vi "Add State (to Connections).vi"(8 "error in (no error)":errorcluster, 10 "State":string, 11 "Channel Ref in":T1 format="%.0x") -> (0 "error out":errorcluster, 3 "Channel Ref out":T1=18446744073709551615 format="%.0x")   [LabVIEW 2017, in "Switch Scripting.lvlib"]
uses:
  Switch Scripting.lvlib
  <vilib>/NI Veristand/Custom Device API/Custom Device Item Ref.ctl
  NationalInstruments.VeriStand.SystemDefinitionAPI
  Shared/Constants.vi
  Shared/Switch Shared.lvlib
  <vilib>/NI VeriStand/Custom Device API/Custom Device API.lvlib
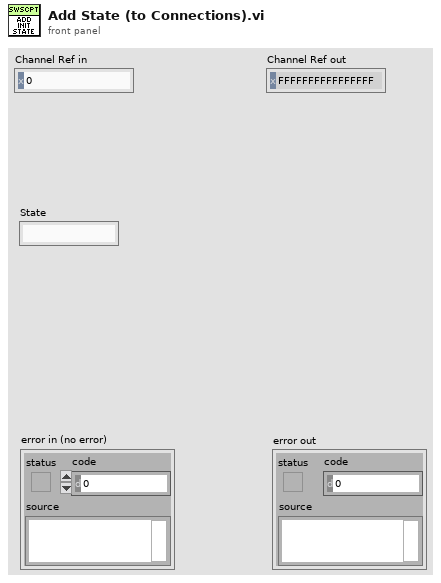
[diagram p1: front panel]
types:
  T1 = typedef "Custom Device API.lvlib/Custom Device Item Ref.ctl" = u64
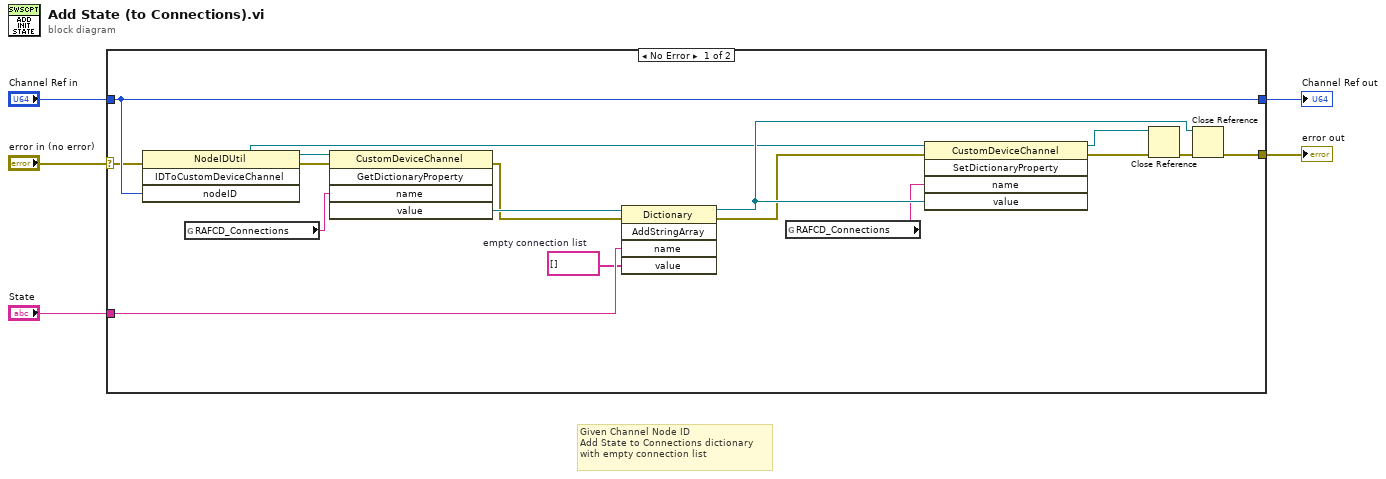
[diagram p0: block diagram]
diagram:
  # "Given Channel Node ID\nAdd State to Connections dictionary\nwith empty connection list"
  n1 = case shown="No Error" "error in (no error)" {
    selector: "error in (no error)" -> [w17 w23]
    tunnel: [w21 w23] -> w4
    tunnel: "Channel Ref in" -> [w18 w22]
    tunnel: [w18 w22] -> w2
    tunnel: "State" -> [w14 _]
    frame No Error {
      w9 = string[] []  # empty connection list
      n2 = invoke class="NodeIDUtil" method="IDToCustomDeviceChannel"(error in=w17, "nodeID"=w18) -> (error out=w19:errorcluster, "IDToCustomDeviceChannel"=w8:refnum<k24>)  [unwired: 2 in, 2 out]
      n3 = global read "Constants.vi" "RAFCD_Connections"() -> (w7:string)
      n4 = invoke class="CustomDeviceChannel" method="GetDictionaryProperty"(reference=w8, error in=w19, "name"=w7) -> (error out=w15:errorcluster, "value"=w16:refnum<k24>)  [unwired: 2 in, 3 out]
      n5 = invoke class="Dictionary" method="AddStringArray"(reference=w16, error in=w15, "name"=w14, "value"=w9) -> (reference out=w13:refnum<k24>, error out=w10:errorcluster)  [unwired: 1 in, 3 out]
      n6 = global read "Constants.vi" "RAFCD_Connections"() -> (w6:string)
      n7 = invoke class="CustomDeviceChannel" method="SetDictionaryProperty"(reference=w8, error in=w10, "name"=w6, "value"=w13) -> (reference out=w11:refnum<k24>, error out=w12:errorcluster)  [unwired: 1 in, 3 out]
      n8 = Close Reference(reference=w11, error in (no error)=w12) -> (error out=w20:errorcluster)
      n9 = Close Reference(reference=w13, error in (no error)=w20) -> (error out=w21:errorcluster)
    }
    frame Error {
    }
  }
  "Channel Ref out" <- w2
  "error out" <- w4
